vi "LED.vi"(2 "LED":cluster{"Red":bool, "Green":bool, "Blue":bool}, 3 "Bot Settings":T1) -> (1 "Bot Settings out":T1)   [LabVIEW 2012]
uses:
  <userlib>/BotSpeak/VIs/Direct/BotSpeak_Control.ctl
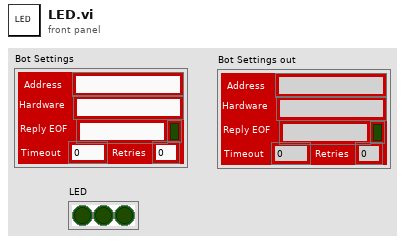
[diagram p1: front panel]
types:
  T1 = typedef "BotSpeak_Control.ctl" = cluster{"Address":string, "Reply EOF":string, "Hardware":string, "Retries":i8, "Timeout":i32, "Open?":bool}
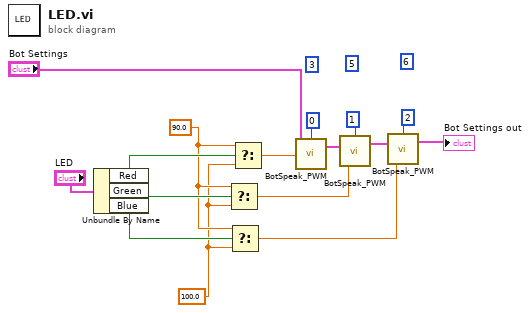
[diagram p0: block diagram]
diagram:
  (unwired) u8 6 ("PWM Line")
  (unwired) u8 5 ("PWM Line")
  (unwired) u8 3 ("PWM Line")
  w3 = 100.0 ("f")
  w4 = 90.0 ("t")
  n1 = Unbundle By Name("LED") -> ("Red"=w10:bool, "Green"=w8:bool, "Blue"=w7:bool)
  n2 = Select(t=w4, s=w8, f=w3) -> (s? t:f=w6:dbl)
  n3 = Select(t=w4, s=w7, f=w3) -> (s? t:f=w5:dbl)
  n4 = Select(t=w4, s=w10, f=w3) -> (s? t:f=w9:dbl)
  n5 = call <userlib>:"BotSpeak_PWM.vi"("Strength (100)"=w9, "Bot Settings"="Bot Settings", "PWM Line"=u8 0) -> ("Bot Settings out"=w15:T1)  [unwired: 1 out]
  n6 = call <userlib>:"BotSpeak_PWM.vi"("Strength (100)"=w6, "Bot Settings"=w15, "PWM Line"=u8 1) -> ("Bot Settings out"=w14:T1)  [unwired: 1 out]
  n7 = call <userlib>:"BotSpeak_PWM.vi"("Strength (100)"=w5, "Bot Settings"=w14, "PWM Line"=u8 2) -> ("Bot Settings out"=→"Bot Settings out":T1)  [unwired: 1 out]
